vi "Inverter Command Write.vi"(0 "GEA2 Reference In":refnum<k24>, 5 "Command Requested":T5, 7 "Command Inputs":T3={"Stop"={"Command Requested"=enum."2 - Stop", "Command Sequence #"=0}, "Closed Loop Spin"={"Command Requested"=enum."4 - Closed Loop", "Command Sequence #"=0, "Closed Loop Ramp Rate"=0, "Closed Loop Target Speed"=0}, "Dry Load Sense"={"Command Requested"=enum."4 - Closed Loop", "Command Sequence #"=0, "Dry Load Ramp Rate 1"=0, "Dry Load Target Speed 1"=0, "Dry Load Dwell Time"=0, "Dry Load Dwell Sample #"=0, "Dry Load Ramp Rate 2"=0, "Dry Load Target Speed 2"=0, "DryLoad Dwell Period(Msec)"=0, "DryLoad Ramp Sample(Msec)"=0}, "Agitate"={"Command Sequence #"=0, "Agitate # of Entries"=0, "Agitate Repeat Count"=0, "Agitate Ramp Rate 1"=0, "Agitate Target Speed 1"=0, "Agitate On Time(Msec) 1"=0, "Agitate Off Time(Msec) 1"=0, "Agitate Ramp Rate 2"=0, "Agitate Target Speed 2"=0, "Agitate On Time(Msec) 2"=0, "Agitate Off Time(Msec) 2"=0, "Agitate Ramp Rate 3"=0, "Agitate Target Speed 3"=0, "Agitate On Time(Msec) 3"=0, "Agitate Off Time(Msec) 3"=0, "Agitate Ramp Rate 4"=0, "Agitate Target Speed 4"=0, "Agitate On Time(Msec) 4"=0, "Agitate Off Time(Msec) 4"=0, "Agitate Ramp Rate 5"=0, "Agitate Target Speed 5"=0, "Agitate On Time(Msec) 5"=0, "Agitate Off Time(Msec) 5"=0, "Agitate Ramp Rate 6"=0, "Agitate Target Speed 6"=0, "Agitate On Time(Msec) 6"=0, "Agitate Off Time(Msec) 6"=0, "Agitate Ramp Rate 7"=0, "Agitate Target Speed 7"=0, "Agitate On Time(Msec) 7"=0, "Agitate Off Time(Msec) 7"=0, "Agitate Ramp Rate 8"=0, "Agitate Target Speed 8"=0, "Agitate On Time(Msec) 8"=0, "Agitate Off Time(Msec) 8"=0, "Agitate Ramp Rate 9"=0, "Agitate Target Speed 9"=0, "Agitate On Time(Msec) 9"=0, "Agitate Off Time(Msec) 9"=0, "Agitate Ramp Rate 10"=0, "Agitate Target Speed 10"=0, "Agitate On Time(Msec) 10"=0, "Agitate Off Time(Msec) 10"=0, "Entry 1"=FALSE, "Entry 2"=FALSE, "Entry 3"=FALSE, "Entry 4"=FALSE, "Entry 5"=FALSE, "Entry 6"=FALSE, "Entry 7"=FALSE, "Entry 8"=FALSE, "Entry 9"=FALSE, "Entry 10"=FALSE, "Command Requested"=enum."3 - Agitate"}, "Open Loop"={"Command Sequence #"=0, "Open Loop # of Entries "=0, "Open Loop Repeat Count"=0, "Open Loop Amplitude % 1"=0, "Open Loop Target Speed 1"=0, "Open Loop On time(Msec) 1"=0, "Open Loop Off Time(Msec) 1"=0, "Open Loop Amplitude % 2"=0, "Open Loop Target Speed 2"=0, "Open Loop On time(Msec) 2"=0, "Open Loop Off Time(Msec) 2"=0, "Open Loop Amplitude % 3"=0, "Open Loop Target Speed 3"=0, "Open Loop On time(Msec) 3"=0, "Open Loop Off Time(Msec) 3"=0, "Open Loop Amplitude % 4"=0, "Open Loop Target Speed 4"=0, "Open Loop On time(Msec) 4"=0, "Open Loop Off Time(Msec) 4"=0, "Open Loop Amplitude % 5"=0, "Open Loop Target Speed 5"=0, "Open Loop On time(Msec) 5"=0, "Open Loop Off Time(Msec) 5"=0, "Open Loop Amplitude % 6"=0, "Open Loop Target Speed 6"=0, "Open Loop On time(Msec) 6"=0, "Open Loop Off Time(Msec) 6"=0, "Open Loop Amplitude % 7"=0, "Open Loop Target Speed 7"=0, "Open Loop On time(Msec) 7"=0, "Open Loop Off Time(Msec) 7"=0, "Open Loop Amplitude % 8"=0, "Open Loop Target Speed 8"=0, "Open Loop On time(Msec) 8"=0, "Open Loop Off Time(Msec) 8"=0, "Open Loop Amplitude % 9"=0, "Open Loop Target Speed 9"=0, "Open Loop On time(Msec) 9"=0, "Open Loop Off Time(Msec) 9"=0, "Open Loop Amplitude % 10"=0, "Open Loop Target Speed 10"=0, "Open Loop On time(Msec) 10"=0, "Open Loop Off Time(Msec) 10"=0, "Entry 1"=FALSE, "Entry 2"=FALSE, "Entry 3"=FALSE, "Entry 4"=FALSE, "Entry 5"=FALSE, "Entry 6"=FALSE, "Entry 7"=FALSE, "Entry 8"=FALSE, "Entry 9"=FALSE, "Entry 10"=FALSE, "Command Requested"=enum."5 - Open Loop"}, "Do Nothing"={"Command Requested"=enum."1 - Do Nothing", "Command Sequence #"=255}, "Invalid Command"={"Command Requested"=enum."0 - Invalid Command", "Command Sequence #"=255}} {"Open Loop"."Open Loop # of Entries" max=10; "Agitate"."Agitate # of Entries" max=10}, 11 "Error In":errorcluster) -> (4 "GEA2 Reference Out":refnum<k24>, 6 "appended array":T1[](array[typedef]) {"ERD Number" format="%.0x"}, 15 "Error Out":errorcluster)   [LabVIEW 2021]
uses:
  D:/Common/LabVIEW GEA2 Toolkit/source/GEA3 DLL Source/GeaCommunication.dll
  Common/LabVIEW GEA2 Toolkit/source/GEA3 DLL Source/GeaCommunication.dll
  Type Defs/Command Requested.ctl
  Type Defs/Command Inputs.ctl
  Laundry Tool (TLMB)/Laundry Tool (TLMB)/Laundry Tool Support/type defs/Inverter_Stop.ctl
  Laundry Tool (TLMB)/Laundry Tool (TLMB)/Laundry Tool Support/type defs/Inverter_Closed_Loop_Spin.ctl
  Laundry Tool (TLMB)/Laundry Tool (TLMB)/Laundry Tool Support/type defs/Inverter_Dry_Load_Sense.ctl
  Laundry Tool (TLMB)/Laundry Tool (TLMB)/Laundry Tool Support/type defs/Inverter_Agitate.ctl
  Laundry Tool (TLMB)/Laundry Tool (TLMB)/Laundry Tool Support/type defs/Inverter_Open_Loop.ctl
  Laundry Tool (TLMB)/Laundry Tool (TLMB)/Laundry Tool Support/type defs/Inverter_Do_Nothing.ctl
  Laundry Tool (TLMB)/Laundry Tool (TLMB)/Laundry Tool Support/type defs/Inverter_Invalid_command.ctl
  Common/LabVIEW GEA2 Toolkit/GEA3/type defs/ERD Write Data In.ctl
  Common/LabVIEW GEA2 Toolkit/GEA3/type defs/Data Type.ctl
  Common/LabVIEW GEA2 Toolkit/GEA3/type defs/Source_Destination.ctl
  Common/LabVIEW GEA2 Toolkit/GEA3/library/GEA2_Toolkit.lvlib
panel:
  in  "Standalone?":bool
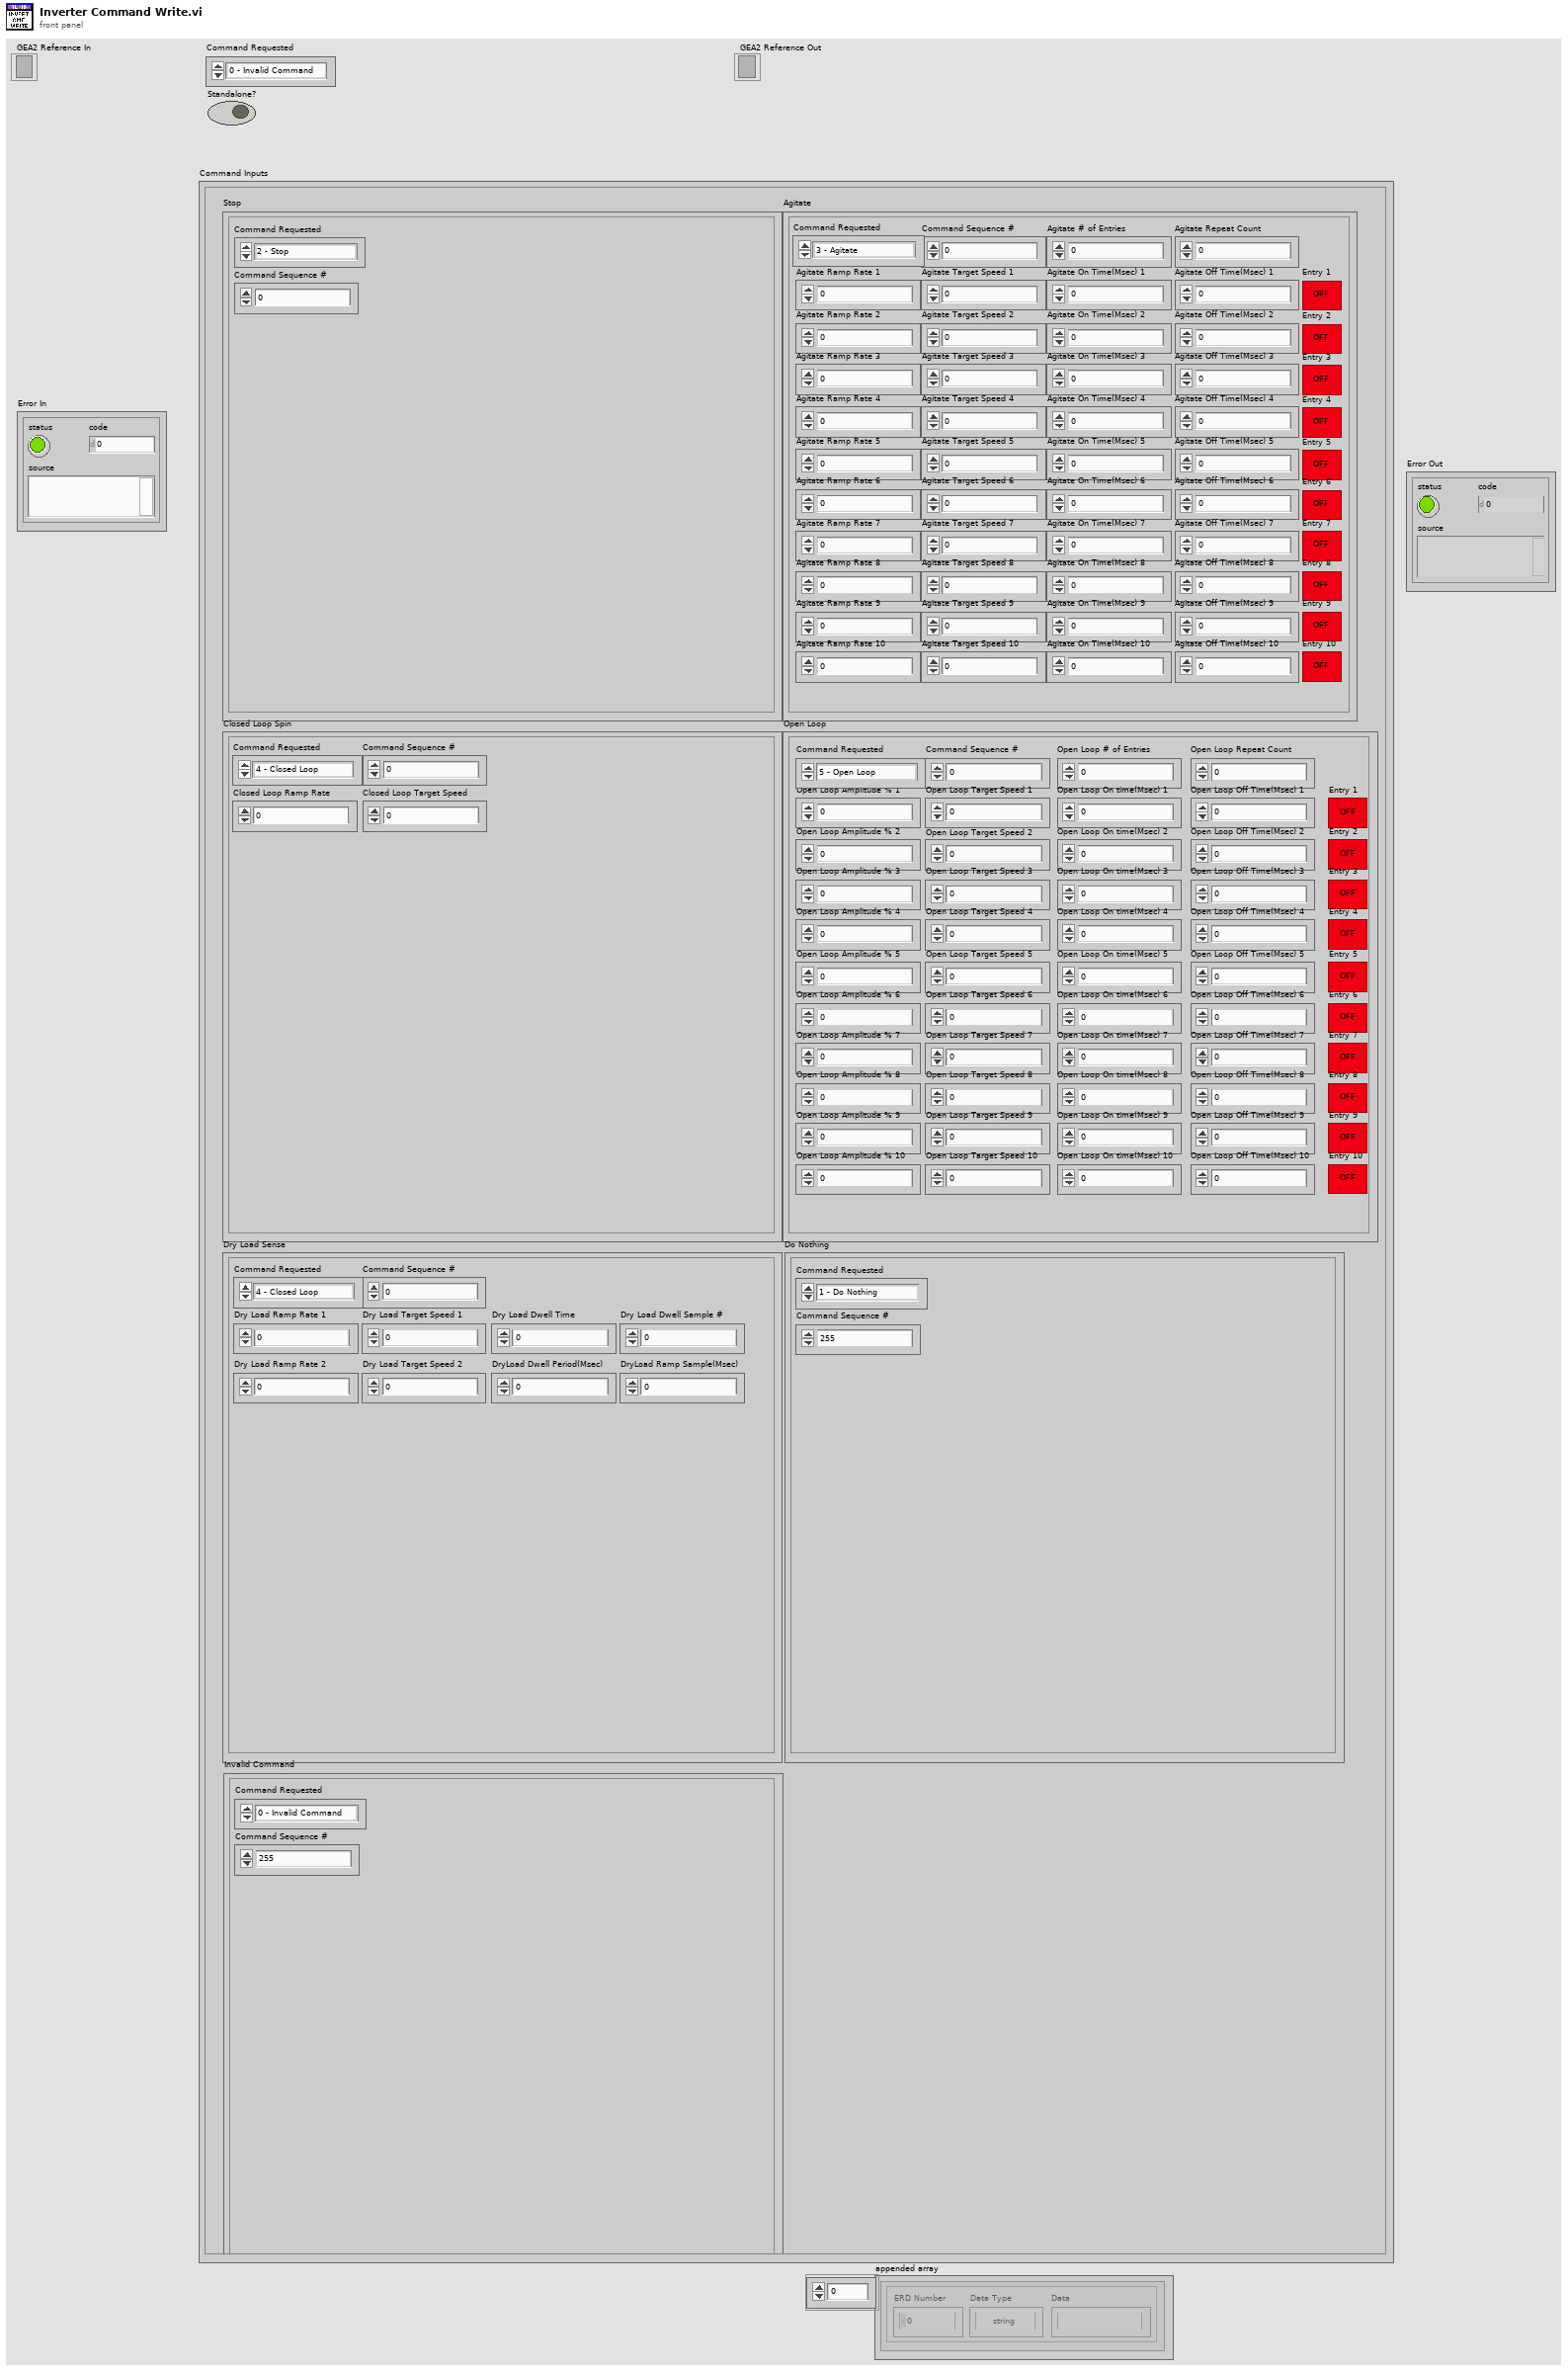
[diagram p1: front panel]
types:
  T1 = typedef "ERD Write Data In.ctl" = cluster{"ERD Number":u16, "Data Type":T2, "Data":string}
  T2 = typedef "Data Type.ctl" = enum16{"string", "boolean", "uint8_t", "uint16_t", "uint32_t", "uint64_t", "int8_t", "int16_t", "int32_t", "int64_t"}
  T3 = typedef "Command Inputs.ctl" = cluster{"Stop":T4, "Closed Loop Spin":T6, "Dry Load Sense":T7, "Agitate":T8, "Open Loop":T9, "Do Nothing":T10, "Invalid Command":T11}
  T4 = typedef "Inverter_Stop.ctl" = cluster{"Command Requested":T5, "Command Sequence #":u8}
  T5 = typedef "Command Requested.ctl" = enum16{"0 - Invalid Command", "1 - Do Nothing", "2 - Stop", "3 - Agitate", "4 - Closed Loop", "5 - Open Loop", "6 - Dry Load Sense"}
  T6 = typedef "Inverter_Closed_Loop_Spin.ctl" = cluster{"Command Requested":T5, "Command Sequence #":u8, "Closed Loop Ramp Rate":u16, "Closed Loop Target Speed":i16}
  T7 = typedef "Inverter_Dry_Load_Sense.ctl" = cluster{"Command Requested":T5, "Command Sequence #":u8, "Dry Load Ramp Rate 1":u16, "Dry Load Target Speed 1":i16, "Dry Load Dwell Time":u16, "Dry Load Dwell Sample #":u16, "Dry Load Ramp Rate 2":u16, "Dry Load Target Speed 2":i16, "DryLoad Dwell Period(Msec)":u16, "DryLoad Ramp Sample(Msec)":u16}
  T8 = typedef "Inverter_Agitate.ctl" = cluster{"Command Sequence #":u8, "Agitate # of Entries":u8, "Agitate Repeat Count":u8, "Agitate Ramp Rate 1":u16, "Agitate Target Speed 1":i16, "Agitate On Time(Msec) 1":u16, "Agitate Off Time(Msec) 1":u16, "Agitate Ramp Rate 2":u16, "Agitate Target Speed 2":i16, "Agitate On Time(Msec) 2":u16, "Agitate Off Time(Msec) 2":u16, "Agitate Ramp Rate 3":u16, "Agitate Target Speed 3":i16, "Agitate On Time(Msec) 3":u16, "Agitate Off Time(Msec) 3":u16, "Agitate Ramp Rate 4":u16, "Agitate Target Speed 4":i16, "Agitate On Time(Msec) 4":u16, "Agitate Off Time(Msec) 4":u16, "Agitate Ramp Rate 5":u16, "Agitate Target Speed 5":i16, "Agitate On Time(Msec) 5":u16, "Agitate Off Time(Msec) 5":u16, "Agitate Ramp Rate 6":u16, "Agitate Target Speed 6":i16, "Agitate On Time(Msec) 6":u16, "Agitate Off Time(Msec) 6":u16, "Agitate Ramp Rate 7":u16, "Agitate Target Speed 7":i16, "Agitate On Time(Msec) 7":u16, "Agitate Off Time(Msec) 7":u16, "Agitate Ramp Rate 8":u16, "Agitate Target Speed 8":i16, "Agitate On Time(Msec) 8":u16, "Agitate Off Time(Msec) 8":u16, "Agitate Ramp Rate 9":u16, "Agitate Target Speed 9":i16, "Agitate On Time(Msec) 9":u16, "Agitate Off Time(Msec) 9":u16, "Agitate Ramp Rate 10":u16, "Agitate Target Speed 10":i16, "Agitate On Time(Msec) 10":u16, "Agitate Off Time(Msec) 10":u16, "Entry 1":bool, "Entry 2":bool, "Entry 3":bool, "Entry 4":bool, "Entry 5":bool, "Entry 6":bool, "Entry 7":bool, "Entry 8":bool, "Entry 9":bool, "Entry 10":bool, "Command Requested":T5}
  T9 = typedef "Inverter_Open_Loop.ctl" = cluster{"Command Sequence #":u8, "Open Loop # of Entries ":u8, "Open Loop Repeat Count":u8, "Open Loop Amplitude % 1":i16, "Open Loop Target Speed 1":i16, "Open Loop On time(Msec) 1":u16, "Open Loop Off Time(Msec) 1":u16, "Open Loop Amplitude % 2":i16, "Open Loop Target Speed 2":i16, "Open Loop On time(Msec) 2":u16, "Open Loop Off Time(Msec) 2":u16, "Open Loop Amplitude % 3":i16, "Open Loop Target Speed 3":i16, "Open Loop On time(Msec) 3":u16, "Open Loop Off Time(Msec) 3":u16, "Open Loop Amplitude % 4":i16, "Open Loop Target Speed 4":i16, "Open Loop On time(Msec) 4":u16, "Open Loop Off Time(Msec) 4":u16, "Open Loop Amplitude % 5":i16, "Open Loop Target Speed 5":i16, "Open Loop On time(Msec) 5":u16, "Open Loop Off Time(Msec) 5":u16, "Open Loop Amplitude % 6":i16, "Open Loop Target Speed 6":i16, "Open Loop On time(Msec) 6":u16, "Open Loop Off Time(Msec) 6":u16, "Open Loop Amplitude % 7":i16, "Open Loop Target Speed 7":i16, "Open Loop On time(Msec) 7":u16, "Open Loop Off Time(Msec) 7":u16, "Open Loop Amplitude % 8":i16, "Open Loop Target Speed 8":i16, "Open Loop On time(Msec) 8":u16, "Open Loop Off Time(Msec) 8":u16, "Open Loop Amplitude % 9":i16, "Open Loop Target Speed 9":i16, "Open Loop On time(Msec) 9":u16, "Open Loop Off Time(Msec) 9":u16, "Open Loop Amplitude % 10":i16, "Open Loop Target Speed 10":i16, "Open Loop On time(Msec) 10":u16, "Open Loop Off Time(Msec) 10":u16, "Entry 1":bool, "Entry 2":bool, "Entry 3":bool, "Entry 4":bool, "Entry 5":bool, "Entry 6":bool, "Entry 7":bool, "Entry 8":bool, "Entry 9":bool, "Entry 10":bool, "Command Requested":T5}
  T10 = typedef "Inverter_Do_Nothing.ctl" = cluster{"Command Requested":T5, "Command Sequence #":u8}
  T11 = typedef "Inverter_Invalid_command.ctl" = cluster{"Command Requested":T5, "Command Sequence #":u8}
  T12 = typedef "Source_Destination.ctl" = cluster{"Source":u8, "Destination":u8}
  T13 = typedef "Data In.ctl" = cluster{"Source":u8, "Destination":u8, "Command":u8, "Message":string}
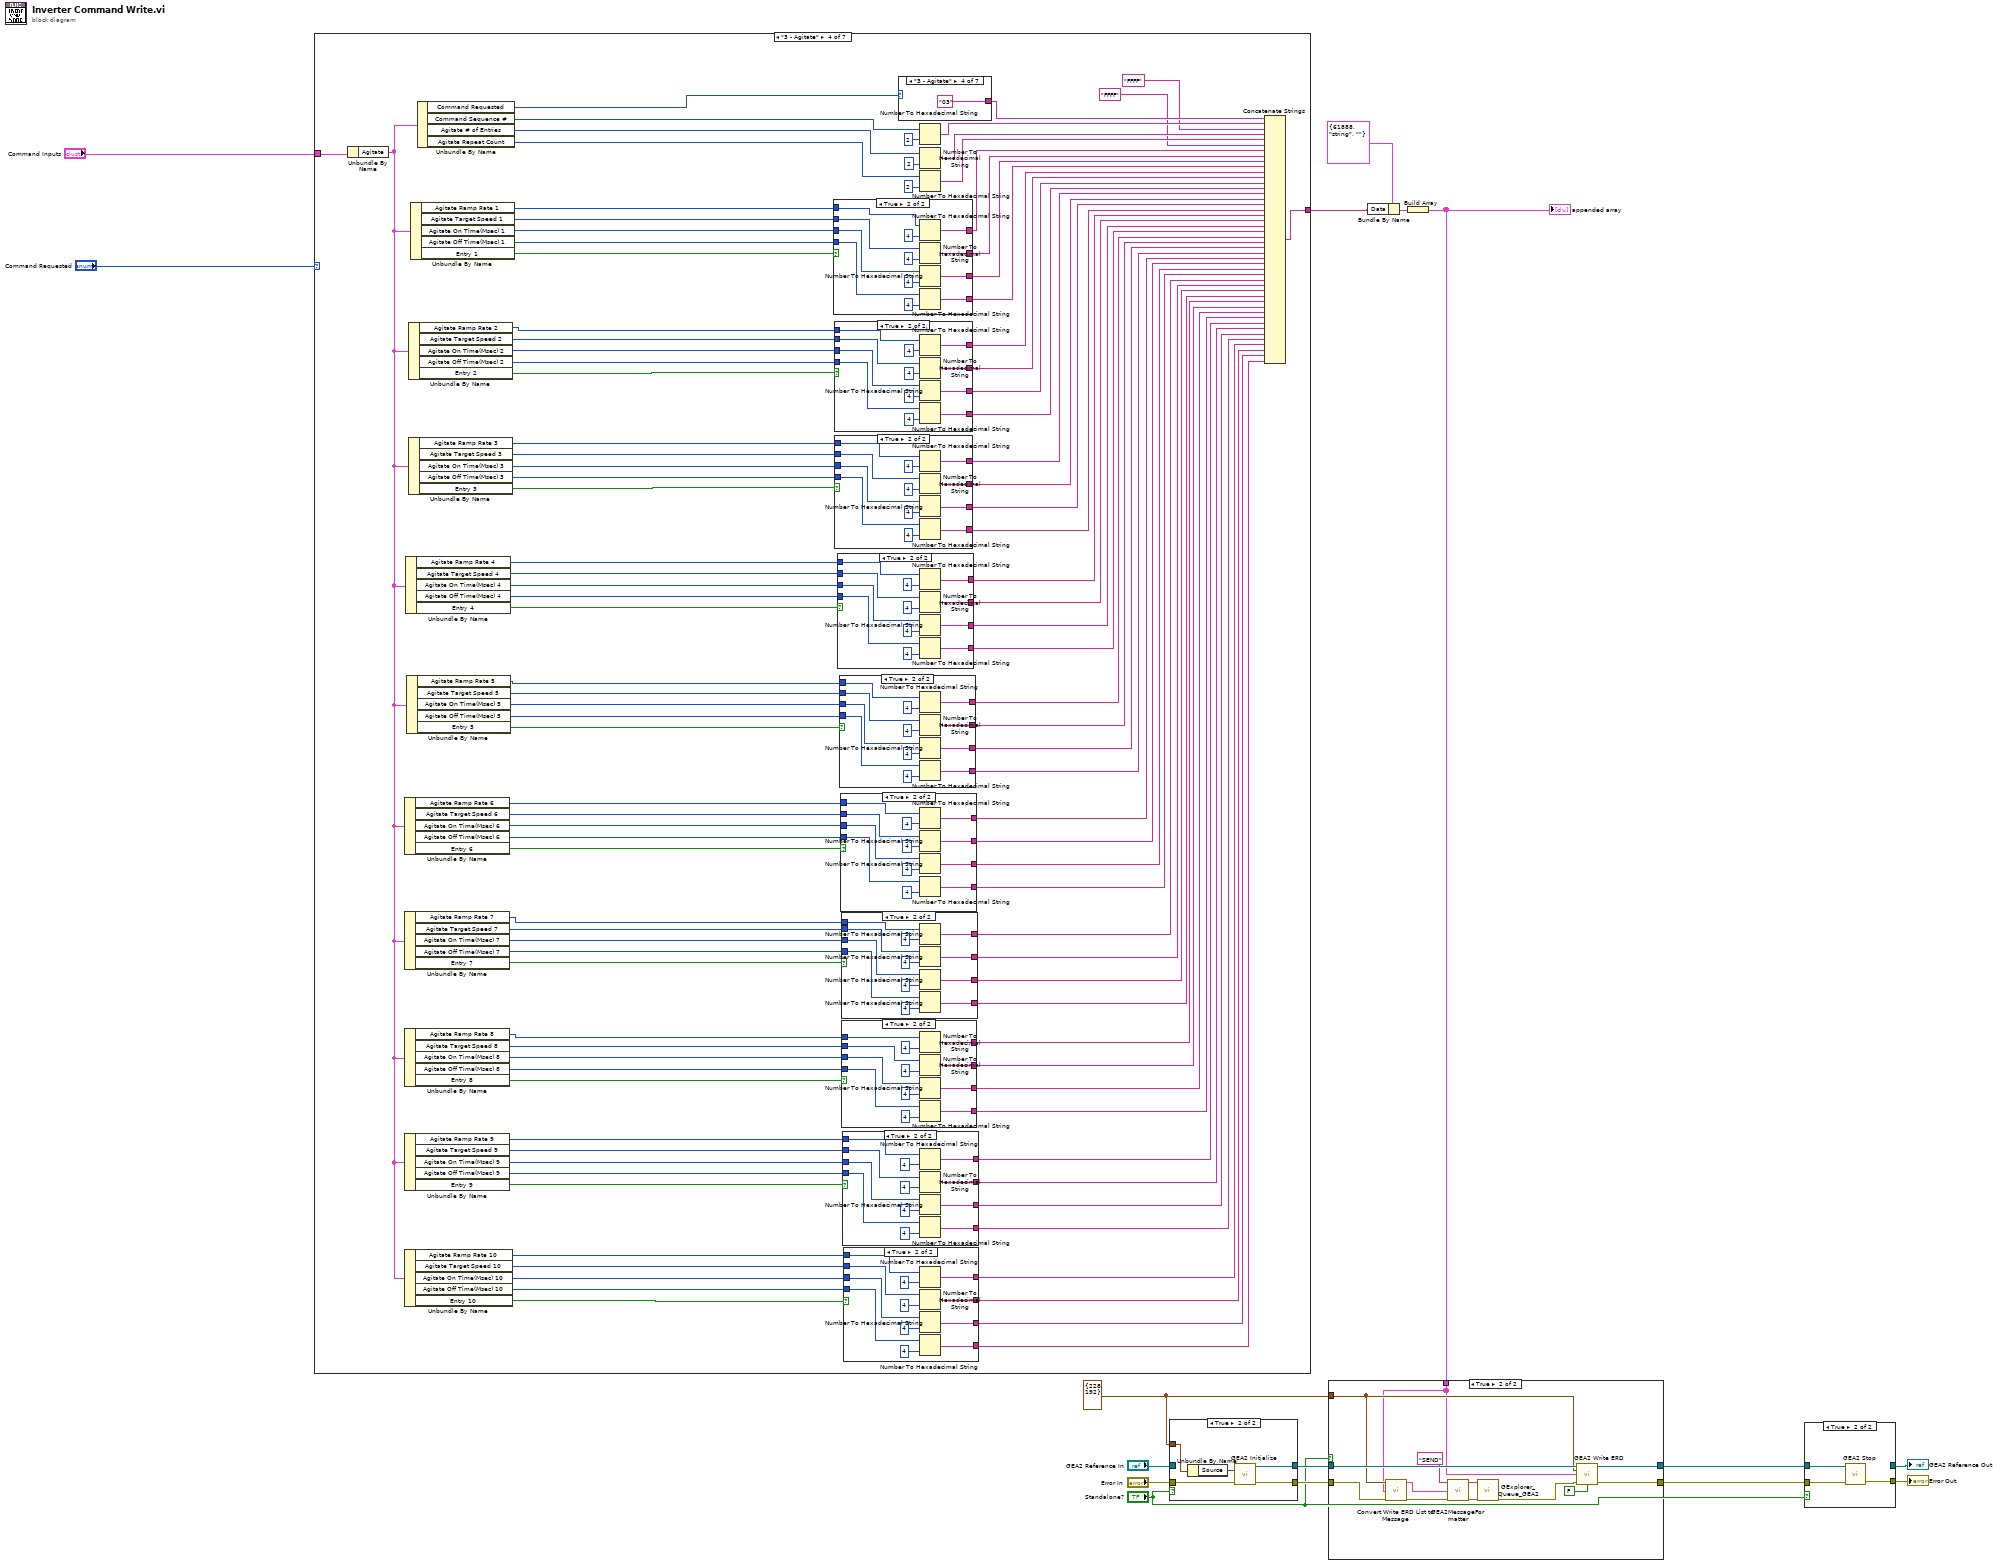
[diagram p0: block diagram]
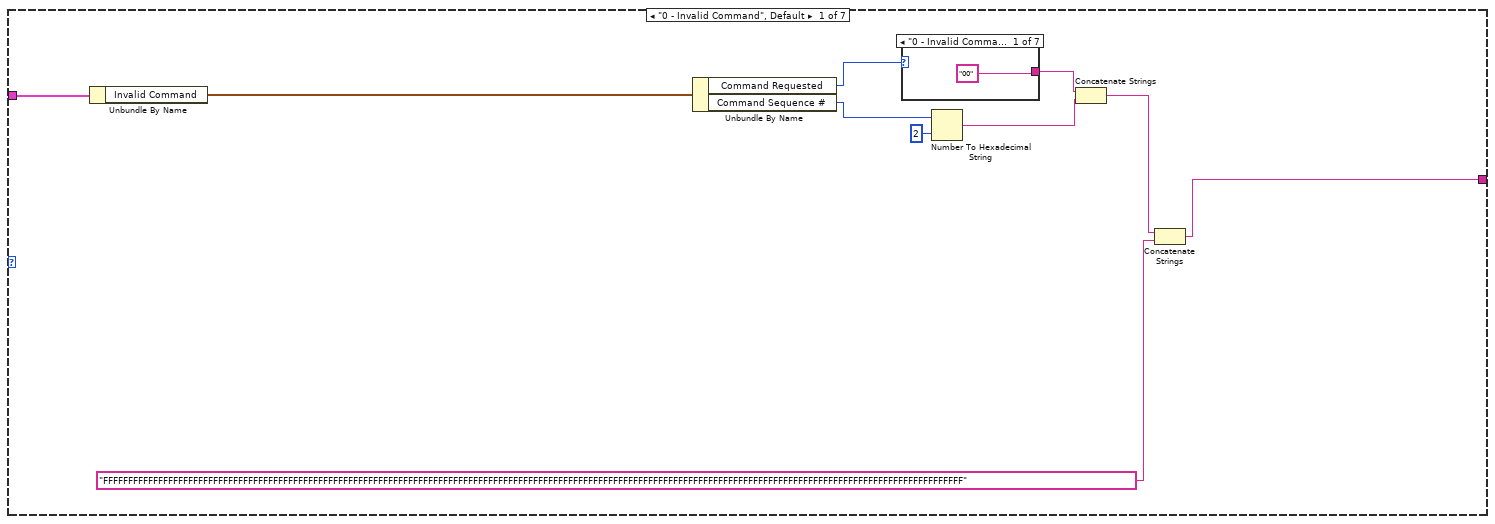
[diagram p5: hidden frame]
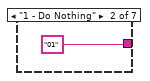
[diagram p6: hidden frame]
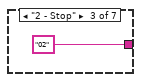
[diagram p7: hidden frame]
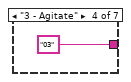
[diagram p8: hidden frame]
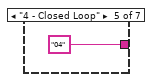
[diagram p9: hidden frame]
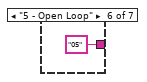
[diagram p10: hidden frame]
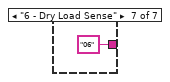
[diagram p11: hidden frame]
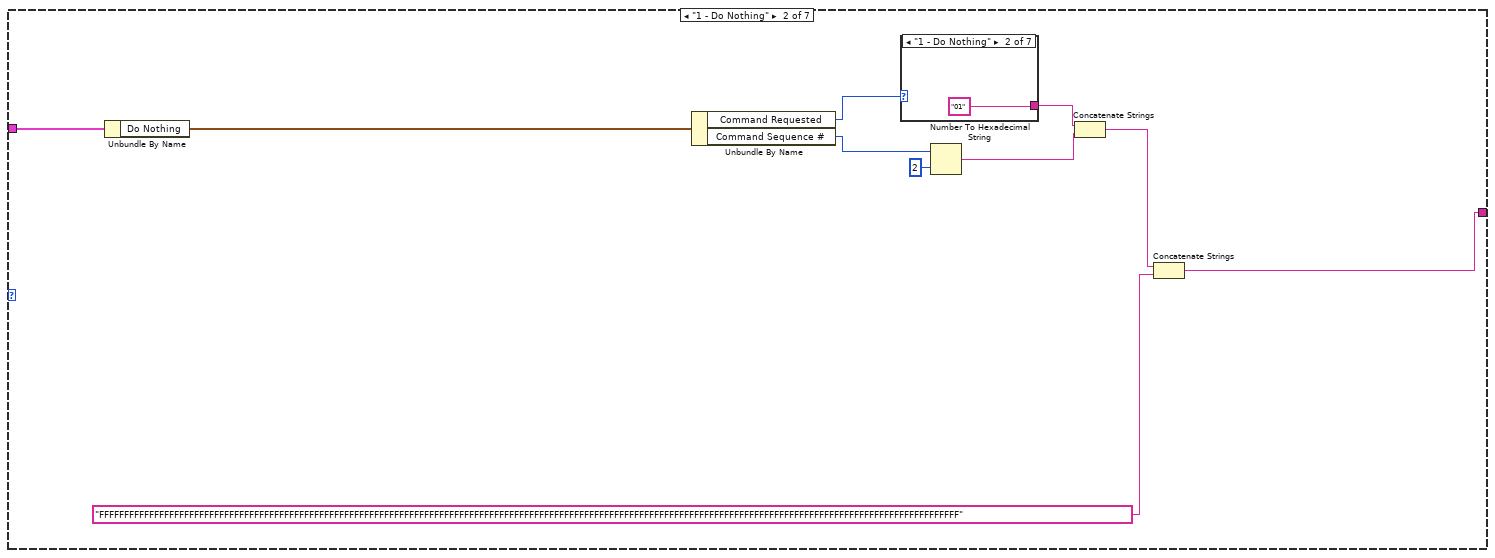
[diagram p12: hidden frame]
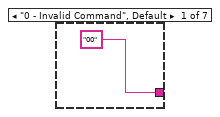
[diagram p13: hidden frame]
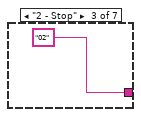
[diagram p14: hidden frame]
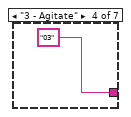
[diagram p15: hidden frame]
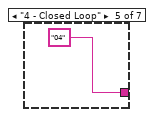
[diagram p16: hidden frame]
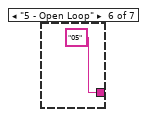
[diagram p17: hidden frame]
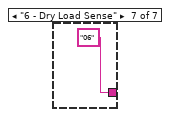
[diagram p18: hidden frame]
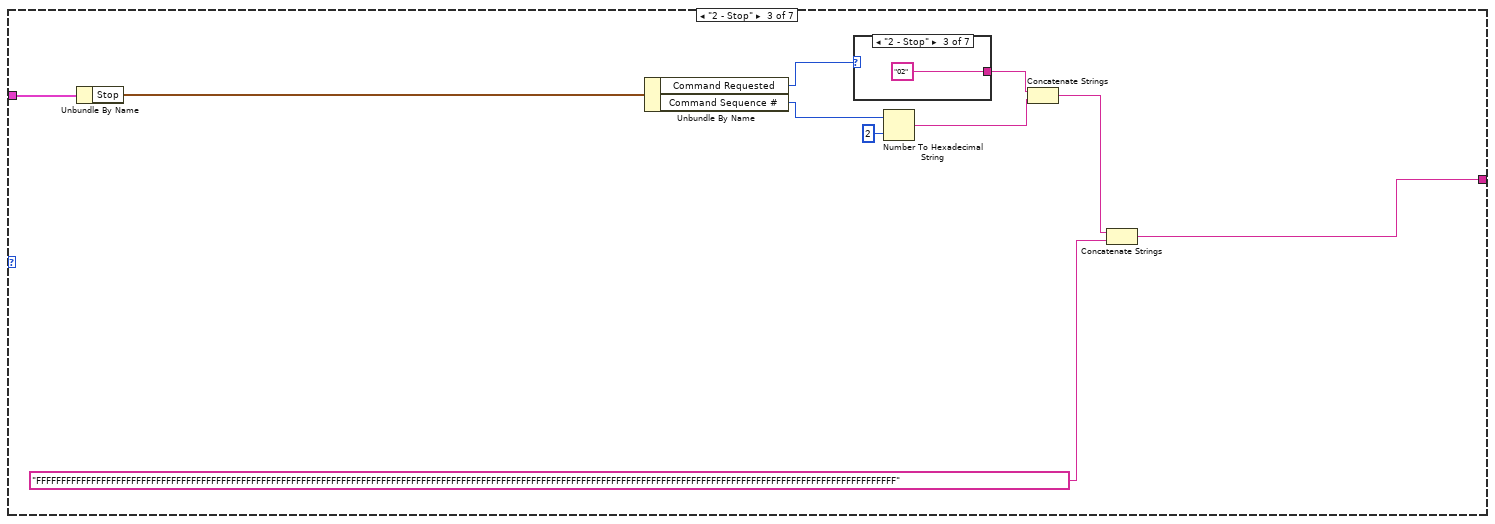
[diagram p19: hidden frame]
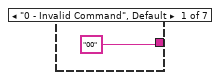
[diagram p20: hidden frame]
diagram:
  w6 = T12 {"Source"=228, "Destination"=192} ("GEA Inputs")
  n1 = case shown="\"3 - Agitate\"" "Command Requested" {
    tunnel: [w17 w34 w51 w121 w341 w415 w637] -> w2
    tunnel: "Command Inputs" -> [w18 w35 w52 w120 w342 w416 w638]
    frame "0 - Invalid Command", Default {
      n2 = Unbundle By Name(w18) -> ("Invalid Command"=w19:T11)
      n3 = Unbundle By Name(w19) -> ("Command Requested"=w26:T5, "Command Sequence #"=w25:u8)
      n4 = case shown="\"0 - Invalid Command\", Default" w26 {
        tunnel: ["00" "01" "02" "03" "04" "05" "06"] -> w23
        frame "0 - Invalid Command", Default {
        }
        frame "1 - Do Nothing" {
        }
        frame "2 - Stop" {
        }
        frame "3 - Agitate" {
        }
        frame "4 - Closed Loop" {
        }
        frame "5 - Open Loop" {
        }
        frame "6 - Dry Load Sense" {
        }
      }
      n5 = Number To Hexadecimal String(1:i16 2 ("width (-)"), 2:w25) -> (0:w22:string)
      n6 = Concatenate Strings(w23, w22) -> (w21:string)
      n7 = Concatenate Strings(w21, "FFFFFFFFFFFFFFFFFFFFFFFFFFFFFFFFFFFFFFFFFFFFFFFFFFFFFFFFFFFFFFFFFFFFFFFFFFFFFFFFFFFFFFFFFFFFFFFFFFFFFFFFFFFFFFFFFFFFFFFFFFFFFFFFFFFFFFFFFFFFFFFFFFFFFFFFFFFFFFFFFFFFFFFFFFFF" ("string")) -> (w17:string)
    }
    frame "1 - Do Nothing" {
      n8 = Unbundle By Name(w35) -> ("Do Nothing"=w36:T10)
      n9 = Unbundle By Name(w36) -> ("Command Requested"=w43:T5, "Command Sequence #"=w42:u8)
      n10 = case shown="\"1 - Do Nothing\"" w43 {
        tunnel: ["00" "01" "02" "03" "04" "05" "06"] -> w40
        frame "0 - Invalid Command", Default {
        }
        frame "1 - Do Nothing" {
        }
        frame "2 - Stop" {
        }
        frame "3 - Agitate" {
        }
        frame "4 - Closed Loop" {
        }
        frame "5 - Open Loop" {
        }
        frame "6 - Dry Load Sense" {
        }
      }
      n11 = Number To Hexadecimal String(1:i16 2 ("width (-)"), 2:w42) -> (0:w39:string)
      n12 = Concatenate Strings(w40, w39) -> (w38:string)
      n13 = Concatenate Strings(w38, "FFFFFFFFFFFFFFFFFFFFFFFFFFFFFFFFFFFFFFFFFFFFFFFFFFFFFFFFFFFFFFFFFFFFFFFFFFFFFFFFFFFFFFFFFFFFFFFFFFFFFFFFFFFFFFFFFFFFFFFFFFFFFFFFFFFFFFFFFFFFFFFFFFFFFFFFFFFFFFFFFFFFFFFFFFFF" ("string")) -> (w34:string)
    }
    frame "2 - Stop" {
      n14 = Unbundle By Name(w52) -> ("Stop"=w53:T4)
      n15 = Unbundle By Name(w53) -> ("Command Requested"=w60:T5, "Command Sequence #"=w59:u8)
      n16 = case shown="\"2 - Stop\"" w60 {
        tunnel: ["00" "01" "02" "03" "04" "05" "06"] -> w57
        frame "0 - Invalid Command", Default {
        }
        frame "1 - Do Nothing" {
        }
        frame "2 - Stop" {
        }
        frame "3 - Agitate" {
        }
        frame "4 - Closed Loop" {
        }
        frame "5 - Open Loop" {
        }
        frame "6 - Dry Load Sense" {
        }
      }
      n17 = Number To Hexadecimal String(1:i16 2 ("width (-)"), 2:w59) -> (0:w56:string)
      n18 = Concatenate Strings(w57, w56) -> (w55:string)
      n19 = Concatenate Strings(w55, "FFFFFFFFFFFFFFFFFFFFFFFFFFFFFFFFFFFFFFFFFFFFFFFFFFFFFFFFFFFFFFFFFFFFFFFFFFFFFFFFFFFFFFFFFFFFFFFFFFFFFFFFFFFFFFFFFFFFFFFFFFFFFFFFFFFFFFFFFFFFFFFFFFFFFFFFFFFFFFFFFFFFFFFFFFFF" ("string")) -> (w51:string)
    }
    frame "3 - Agitate" {
      n20 = Unbundle By Name(w120) -> ("Agitate"=w68:T8)
      n21 = Unbundle By Name(w68) -> ("Agitate Ramp Rate 10"=w72:u16, "Agitate Target Speed 10"=w71:i16, "Agitate On Time(Msec) 10"=w70:u16, "Agitate Off Time(Msec) 10"=w69:u16, "Entry 10"=w105:bool)
      n22 = Unbundle By Name(w68) -> ("Agitate Ramp Rate 6"=w88:u16, "Agitate Target Speed 6"=w87:i16, "Agitate On Time(Msec) 6"=w86:u16, "Agitate Off Time(Msec) 6"=w85:u16, "Entry 6"=w109:bool)
      n23 = Unbundle By Name(w68) -> ("Agitate Ramp Rate 7"=w84:u16, "Agitate Target Speed 7"=w83:i16, "Agitate On Time(Msec) 7"=w82:u16, "Agitate Off Time(Msec) 7"=w81:u16, "Entry 7"=w108:bool)
      n24 = Unbundle By Name(w68) -> ("Agitate Ramp Rate 8"=w80:u16, "Agitate Target Speed 8"=w79:i16, "Agitate On Time(Msec) 8"=w78:u16, "Agitate Off Time(Msec) 8"=w77:u16, "Entry 8"=w107:bool)
      n25 = Unbundle By Name(w68) -> ("Agitate Ramp Rate 9"=w76:u16, "Agitate Target Speed 9"=w75:i16, "Agitate On Time(Msec) 9"=w74:u16, "Agitate Off Time(Msec) 9"=w73:u16, "Entry 9"=w106:bool)
      n26 = Unbundle By Name(w68) -> ("Agitate Ramp Rate 4"=w96:u16, "Agitate Target Speed 4"=w95:i16, "Agitate On Time(Msec) 4"=w94:u16, "Agitate Off Time(Msec) 4"=w93:u16, "Entry 4"=w111:bool)
      n27 = Unbundle By Name(w68) -> ("Agitate Ramp Rate 5"=w92:u16, "Agitate Target Speed 5"=w91:i16, "Agitate On Time(Msec) 5"=w90:u16, "Agitate Off Time(Msec) 5"=w89:u16, "Entry 5"=w110:bool)
      n28 = Unbundle By Name(w68) -> ("Agitate Ramp Rate 2"=w104:u16, "Agitate Target Speed 2"=w103:i16, "Agitate On Time(Msec) 2"=w102:u16, "Agitate Off Time(Msec) 2"=w101:u16, "Entry 2"=w113:bool)
      n29 = Unbundle By Name(w68) -> ("Agitate Ramp Rate 3"=w100:u16, "Agitate Target Speed 3"=w99:i16, "Agitate On Time(Msec) 3"=w98:u16, "Agitate Off Time(Msec) 3"=w97:u16, "Entry 3"=w112:bool)
      n30 = Unbundle By Name(w68) -> ("Agitate Ramp Rate 1"=w117:u16, "Agitate Target Speed 1"=w116:i16, "Agitate On Time(Msec) 1"=w115:u16, "Agitate Off Time(Msec) 1"=w114:u16, "Entry 1"=w118:bool)
      n31 = Unbundle By Name(w68) -> ("Command Requested"=w172:T5, "Command Sequence #"=w171:u8, "Agitate # of Entries"=w167:u8, "Agitate Repeat Count"=w119:u8)
      n32 = case shown="True" w118 {
        tunnel: ["FFFF" w329] -> w161
        tunnel: ["FFFF" w328] -> w160
        tunnel: ["FFFF" w327] -> w159
        tunnel: ["FFFF" w326] -> w158
        tunnel: w117 -> [_ w325]
        tunnel: w116 -> [_ w324]
        tunnel: w115 -> [_ w323]
        tunnel: w114 -> [_ w322]
        frame False {
        }
        frame True {
          n33 = Number To Hexadecimal String(1:i16 4 ("width (-)"), 2:w325) -> (0:w329:string)
          n34 = Number To Hexadecimal String(1:i16 4 ("width (-)"), 2:w324) -> (0:w328:string)
          n35 = Number To Hexadecimal String(1:i16 4 ("width (-)"), 2:w323) -> (0:w327:string)
          n36 = Number To Hexadecimal String(1:i16 4 ("width (-)"), 2:w322) -> (0:w326:string)
        }
      }
      n37 = case shown="True" w113 {
        tunnel: ["FFFF" w313] -> w157
        tunnel: ["FFFF" w312] -> w156
        tunnel: ["FFFF" w311] -> w155
        tunnel: ["FFFF" w310] -> w154
        tunnel: w104 -> [_ w309]
        tunnel: w103 -> [_ w308]
        tunnel: w102 -> [_ w307]
        tunnel: w101 -> [_ w306]
        frame False {
        }
        frame True {
          n38 = Number To Hexadecimal String(1:i16 4 ("width (-)"), 2:w309) -> (0:w313:string)
          n39 = Number To Hexadecimal String(1:i16 4 ("width (-)"), 2:w308) -> (0:w312:string)
          n40 = Number To Hexadecimal String(1:i16 4 ("width (-)"), 2:w307) -> (0:w311:string)
          n41 = Number To Hexadecimal String(1:i16 4 ("width (-)"), 2:w306) -> (0:w310:string)
        }
      }
      n42 = case shown="True" w112 {
        tunnel: ["FFFF" w297] -> w153
        tunnel: ["FFFF" w296] -> w152
        tunnel: ["FFFF" w295] -> w151
        tunnel: ["FFFF" w294] -> w150
        tunnel: w100 -> [_ w293]
        tunnel: w99 -> [_ w292]
        tunnel: w98 -> [_ w291]
        tunnel: w97 -> [_ w290]
        frame False {
        }
        frame True {
          n43 = Number To Hexadecimal String(1:i16 4 ("width (-)"), 2:w293) -> (0:w297:string)
          n44 = Number To Hexadecimal String(1:i16 4 ("width (-)"), 2:w292) -> (0:w296:string)
          n45 = Number To Hexadecimal String(1:i16 4 ("width (-)"), 2:w291) -> (0:w295:string)
          n46 = Number To Hexadecimal String(1:i16 4 ("width (-)"), 2:w290) -> (0:w294:string)
        }
      }
      n47 = case shown="True" w111 {
        tunnel: ["FFFF" w281] -> w149
        tunnel: ["FFFF" w280] -> w148
        tunnel: ["FFFF" w279] -> w147
        tunnel: ["FFFF" w278] -> w146
        tunnel: w96 -> [_ w277]
        tunnel: w95 -> [_ w276]
        tunnel: w94 -> [_ w275]
        tunnel: w93 -> [_ w274]
        frame False {
        }
        frame True {
          n48 = Number To Hexadecimal String(1:i16 4 ("width (-)"), 2:w277) -> (0:w281:string)
          n49 = Number To Hexadecimal String(1:i16 4 ("width (-)"), 2:w276) -> (0:w280:string)
          n50 = Number To Hexadecimal String(1:i16 4 ("width (-)"), 2:w275) -> (0:w279:string)
          n51 = Number To Hexadecimal String(1:i16 4 ("width (-)"), 2:w274) -> (0:w278:string)
        }
      }
      n52 = case shown="True" w110 {
        tunnel: ["FFFF" w265] -> w145
        tunnel: ["FFFF" w264] -> w144
        tunnel: ["FFFF" w263] -> w143
        tunnel: ["FFFF" w262] -> w142
        tunnel: w92 -> [_ w261]
        tunnel: w91 -> [_ w260]
        tunnel: w90 -> [_ w259]
        tunnel: w89 -> [_ w258]
        frame False {
        }
        frame True {
          n53 = Number To Hexadecimal String(1:i16 4 ("width (-)"), 2:w261) -> (0:w265:string)
          n54 = Number To Hexadecimal String(1:i16 4 ("width (-)"), 2:w260) -> (0:w264:string)
          n55 = Number To Hexadecimal String(1:i16 4 ("width (-)"), 2:w259) -> (0:w263:string)
          n56 = Number To Hexadecimal String(1:i16 4 ("width (-)"), 2:w258) -> (0:w262:string)
        }
      }
      n57 = case shown="True" w109 {
        tunnel: ["FFFF" w249] -> w141
        tunnel: ["FFFF" w248] -> w140
        tunnel: ["FFFF" w247] -> w139
        tunnel: ["FFFF" w246] -> w138
        tunnel: w88 -> [_ w245]
        tunnel: w87 -> [_ w244]
        tunnel: w86 -> [_ w243]
        tunnel: w85 -> [_ w242]
        frame False {
        }
        frame True {
          n58 = Number To Hexadecimal String(1:i16 4 ("width (-)"), 2:w245) -> (0:w249:string)
          n59 = Number To Hexadecimal String(1:i16 4 ("width (-)"), 2:w244) -> (0:w248:string)
          n60 = Number To Hexadecimal String(1:i16 4 ("width (-)"), 2:w243) -> (0:w247:string)
          n61 = Number To Hexadecimal String(1:i16 4 ("width (-)"), 2:w242) -> (0:w246:string)
        }
      }
      n62 = case shown="True" w108 {
        tunnel: ["FFFF" w233] -> w137
        tunnel: ["FFFF" w232] -> w136
        tunnel: ["FFFF" w231] -> w135
        tunnel: ["FFFF" w230] -> w134
        tunnel: w84 -> [_ w229]
        tunnel: w83 -> [_ w228]
        tunnel: w82 -> [_ w227]
        tunnel: w81 -> [_ w226]
        frame False {
        }
        frame True {
          n63 = Number To Hexadecimal String(1:i16 4 ("width (-)"), 2:w229) -> (0:w233:string)
          n64 = Number To Hexadecimal String(1:i16 4 ("width (-)"), 2:w228) -> (0:w232:string)
          n65 = Number To Hexadecimal String(1:i16 4 ("width (-)"), 2:w227) -> (0:w231:string)
          n66 = Number To Hexadecimal String(1:i16 4 ("width (-)"), 2:w226) -> (0:w230:string)
        }
      }
      n67 = case shown="True" w107 {
        tunnel: ["FFFF" w217] -> w133
        tunnel: ["FFFF" w216] -> w132
        tunnel: ["FFFF" w215] -> w131
        tunnel: ["FFFF" w214] -> w130
        tunnel: w80 -> [_ w213]
        tunnel: w79 -> [_ w212]
        tunnel: w78 -> [_ w211]
        tunnel: w77 -> [_ w210]
        frame False {
        }
        frame True {
          n68 = Number To Hexadecimal String(1:i16 4 ("width (-)"), 2:w213) -> (0:w217:string)
          n69 = Number To Hexadecimal String(1:i16 4 ("width (-)"), 2:w212) -> (0:w216:string)
          n70 = Number To Hexadecimal String(1:i16 4 ("width (-)"), 2:w211) -> (0:w215:string)
          n71 = Number To Hexadecimal String(1:i16 4 ("width (-)"), 2:w210) -> (0:w214:string)
        }
      }
      n72 = case shown="True" w106 {
        tunnel: ["FFFF" w201] -> w129
        tunnel: ["FFFF" w200] -> w128
        tunnel: ["FFFF" w199] -> w127
        tunnel: ["FFFF" w198] -> w126
        tunnel: w76 -> [_ w197]
        tunnel: w75 -> [_ w196]
        tunnel: w74 -> [_ w195]
        tunnel: w73 -> [_ w194]
        frame False {
        }
        frame True {
          n73 = Number To Hexadecimal String(1:i16 4 ("width (-)"), 2:w197) -> (0:w201:string)
          n74 = Number To Hexadecimal String(1:i16 4 ("width (-)"), 2:w196) -> (0:w200:string)
          n75 = Number To Hexadecimal String(1:i16 4 ("width (-)"), 2:w195) -> (0:w199:string)
          n76 = Number To Hexadecimal String(1:i16 4 ("width (-)"), 2:w194) -> (0:w198:string)
        }
      }
      n77 = case shown="True" w105 {
        tunnel: ["FFFF" w185] -> w125
        tunnel: ["FFFF" w184] -> w124
        tunnel: ["FFFF" w183] -> w123
        tunnel: ["FFFF" w182] -> w122
        tunnel: w72 -> [_ w181]
        tunnel: w71 -> [_ w180]
        tunnel: w70 -> [_ w179]
        tunnel: w69 -> [_ w178]
        frame False {
        }
        frame True {
          n78 = Number To Hexadecimal String(1:i16 4 ("width (-)"), 2:w181) -> (0:w185:string)
          n79 = Number To Hexadecimal String(1:i16 4 ("width (-)"), 2:w180) -> (0:w184:string)
          n80 = Number To Hexadecimal String(1:i16 4 ("width (-)"), 2:w179) -> (0:w183:string)
          n81 = Number To Hexadecimal String(1:i16 4 ("width (-)"), 2:w178) -> (0:w182:string)
        }
      }
      n82 = case shown="\"3 - Agitate\"" w172 {
        tunnel: ["00" "01" "02" "03" "04" "05" "06"] -> w170
        frame "0 - Invalid Command", Default {
        }
        frame "1 - Do Nothing" {
        }
        frame "2 - Stop" {
        }
        frame "3 - Agitate" {
        }
        frame "4 - Closed Loop" {
        }
        frame "5 - Open Loop" {
        }
        frame "6 - Dry Load Sense" {
        }
      }
      n83 = Number To Hexadecimal String(1:i16 2 ("width (-)"), 2:w171) -> (0:w169:string)
      n84 = Number To Hexadecimal String(1:i16 2 ("width (-)"), 2:w167) -> (0:w165:string)
      n85 = Number To Hexadecimal String(1:i16 2 ("width (-)"), 2:w119) -> (0:w163:string)
      n86 = Concatenate Strings(w170, w169, "FFFF" ("string"), w165, w163, "FFFF" ("string"), w161, w160, w159, w158, w157, w156, w155, w154, w153, w152, w151, w150, w149, w148, w147, w146, w145, w144, w143, w142, w141, w140, w139, w138, w137, w136, w135, w134, w133, w132, w131, w130, w129, w128, w127, w126, w125, w124, w123, w122) -> (w121:string)
    }
    frame "4 - Closed Loop" {
      n87 = Unbundle By Name(w342) -> ("Closed Loop Spin"=w346:T6)
      n88 = Unbundle By Name(w346) -> ("Command Requested"=w356:T5, "Command Sequence #"=w354:u8, "Closed Loop Ramp Rate"=w344:u16, "Closed Loop Target Speed"=w349:i16)
      n89 = case shown="\"4 - Closed Loop\"" w356 {
        tunnel: ["00" "01" "02" "03" "04" "05" "06"] -> w355
        frame "0 - Invalid Command", Default {
        }
        frame "1 - Do Nothing" {
        }
        frame "2 - Stop" {
        }
        frame "3 - Agitate" {
        }
        frame "4 - Closed Loop" {
        }
        frame "5 - Open Loop" {
        }
        frame "6 - Dry Load Sense" {
        }
      }
      n90 = Number To Hexadecimal String(1:i16 2 ("width (-)"), 2:w354) -> (0:w352:string)
      n91 = Number To Hexadecimal String(1:i16 4 ("width (-)"), 2:w344) -> (0:w345:string)
      n92 = Number To Hexadecimal String(1:i16 4 ("width (-)"), 2:w349) -> (0:w348:string)
      n93 = Concatenate Strings(w355, w352, "FFFF" ("string"), w345, w348, "FFFFFFFFFFFFFFFFFFFFFFFFFFFFFFFFFFFFFFFFFFFFFFFFFFFFFFFFFFFFFFFFFFFFFFFFFFFFFFFFFFFFFFFFFFFFFFFFFFFFFFFFFFFFFFFFFFFFFFFFFFFFFFFFFFFFFFFFFFFFFFFFFFFFFFFFFFFFFFFF") -> (w341:string)
    }
    frame "5 - Open Loop" {
      n94 = Unbundle By Name(w416) -> ("Open Loop"=w414:T9)
      n95 = Unbundle By Name(w414) -> ("Command Requested"=w466:T5, "Command Sequence #"=w465:u8, "Open Loop # of Entries"=w461:u8, "Open Loop Repeat Count"=w460:u8)
      n96 = Unbundle By Name(w414) -> ("Open Loop Amplitude % 1"=w403:i16, "Open Loop Target Speed 1"=w402:i16, "Open Loop On time(Msec) 1"=w401:u16, "Open Loop Off Time(Msec) 1"=w400:u16, "Entry 1"=w413:bool)
      n97 = Unbundle By Name(w414) -> ("Open Loop Amplitude % 2"=w399:i16, "Open Loop Target Speed 2"=w398:i16, "Open Loop On time(Msec) 2"=w397:u16, "Open Loop Off Time(Msec) 2"=w396:u16, "Entry 2"=w412:bool)
      n98 = Unbundle By Name(w414) -> ("Open Loop Amplitude % 3"=w395:i16, "Open Loop Target Speed 3"=w394:i16, "Open Loop On time(Msec) 3"=w393:u16, "Open Loop Off Time(Msec) 3"=w392:u16, "Entry 3"=w411:bool)
      n99 = Unbundle By Name(w414) -> ("Open Loop Amplitude % 4"=w391:i16, "Open Loop Target Speed 4"=w390:i16, "Open Loop On time(Msec) 4"=w389:u16, "Open Loop Off Time(Msec) 4"=w388:u16, "Entry 4"=w410:bool)
      n100 = Unbundle By Name(w414) -> ("Open Loop Amplitude % 5"=w387:i16, "Open Loop Target Speed 5"=w386:i16, "Open Loop On time(Msec) 5"=w385:u16, "Open Loop Off Time(Msec) 5"=w384:u16, "Entry 5"=w409:bool)
      n101 = Unbundle By Name(w414) -> ("Open Loop Amplitude % 6"=w383:i16, "Open Loop Target Speed 6"=w382:i16, "Open Loop On time(Msec) 6"=w381:u16, "Open Loop Off Time(Msec) 6"=w380:u16, "Entry 6"=w408:bool)
      n102 = Unbundle By Name(w414) -> ("Open Loop Amplitude % 7"=w379:i16, "Open Loop Target Speed 7"=w378:i16, "Open Loop On time(Msec) 7"=w377:u16, "Open Loop Off Time(Msec) 7"=w376:u16, "Entry 7"=w407:bool)
      n103 = Unbundle By Name(w414) -> ("Open Loop Amplitude % 8"=w375:i16, "Open Loop Target Speed 8"=w374:i16, "Open Loop On time(Msec) 8"=w373:u16, "Open Loop Off Time(Msec) 8"=w372:u16, "Entry 8"=w406:bool)
      n104 = Unbundle By Name(w414) -> ("Open Loop Amplitude % 9"=w371:i16, "Open Loop Target Speed 9"=w370:i16, "Open Loop On time(Msec) 9"=w369:u16, "Open Loop Off Time(Msec) 9"=w368:u16, "Entry 9"=w405:bool)
      n105 = Unbundle By Name(w414) -> ("Open Loop Amplitude % 10"=w367:i16, "Open Loop Target Speed 10"=w366:i16, "Open Loop On time(Msec) 10"=w365:u16, "Open Loop Off Time(Msec) 10"=w364:u16, "Entry 10"=w404:bool)
      n106 = case shown="True" w412 {
        tunnel: ["FFFF" w609] -> w452
        tunnel: ["FFFF" w608] -> w451
        tunnel: ["FFFF" w607] -> w450
        tunnel: ["FFFF" w606] -> w449
        tunnel: w399 -> [_ w605]
        tunnel: w398 -> [_ w604]
        tunnel: w397 -> [_ w603]
        tunnel: w396 -> [_ w602]
        frame False {
        }
        frame True {
          n107 = Number To Hexadecimal String(1:i16 4 ("width (-)"), 2:w605) -> (0:w609:string)
          n108 = Number To Hexadecimal String(1:i16 4 ("width (-)"), 2:w604) -> (0:w608:string)
          n109 = Number To Hexadecimal String(1:i16 4 ("width (-)"), 2:w603) -> (0:w607:string)
          n110 = Number To Hexadecimal String(1:i16 4 ("width (-)"), 2:w602) -> (0:w606:string)
        }
      }
      n111 = case shown="True" w413 {
        tunnel: ["FFFF" w625] -> w456
        tunnel: ["FFFF" w624] -> w455
        tunnel: ["FFFF" w623] -> w454
        tunnel: ["FFFF" w622] -> w453
        tunnel: w403 -> [_ w621]
        tunnel: w402 -> [_ w620]
        tunnel: w401 -> [_ w619]
        tunnel: w400 -> [_ w618]
        frame False {
        }
        frame True {
          n112 = Number To Hexadecimal String(1:i16 4 ("width (-)"), 2:w621) -> (0:w625:string)
          n113 = Number To Hexadecimal String(1:i16 4 ("width (-)"), 2:w620) -> (0:w624:string)
          n114 = Number To Hexadecimal String(1:i16 4 ("width (-)"), 2:w619) -> (0:w623:string)
          n115 = Number To Hexadecimal String(1:i16 4 ("width (-)"), 2:w618) -> (0:w622:string)
        }
      }
      n116 = case shown="True" w411 {
        tunnel: ["FFFF" w593] -> w448
        tunnel: ["FFFF" w592] -> w447
        tunnel: ["FFFF" w591] -> w446
        tunnel: ["FFFF" w590] -> w445
        tunnel: w395 -> [_ w589]
        tunnel: w394 -> [_ w588]
        tunnel: w393 -> [_ w587]
        tunnel: w392 -> [_ w586]
        frame False {
        }
        frame True {
          n117 = Number To Hexadecimal String(1:i16 4 ("width (-)"), 2:w589) -> (0:w593:string)
          n118 = Number To Hexadecimal String(1:i16 4 ("width (-)"), 2:w588) -> (0:w592:string)
          n119 = Number To Hexadecimal String(1:i16 4 ("width (-)"), 2:w587) -> (0:w591:string)
          n120 = Number To Hexadecimal String(1:i16 4 ("width (-)"), 2:w586) -> (0:w590:string)
        }
      }
      n121 = case shown="False" w410 {
        tunnel: ["FFFF" w577] -> w444
        tunnel: ["FFFF" w576] -> w443
        tunnel: ["FFFF" w575] -> w442
        tunnel: ["FFFF" w574] -> w441
        tunnel: w391 -> [_ w573]
        tunnel: w390 -> [_ w572]
        tunnel: w389 -> [_ w571]
        tunnel: w388 -> [_ w570]
        frame False {
        }
        frame True {
          n122 = Number To Hexadecimal String(1:i16 4 ("width (-)"), 2:w573) -> (0:w577:string)
          n123 = Number To Hexadecimal String(1:i16 4 ("width (-)"), 2:w572) -> (0:w576:string)
          n124 = Number To Hexadecimal String(1:i16 4 ("width (-)"), 2:w571) -> (0:w575:string)
          n125 = Number To Hexadecimal String(1:i16 4 ("width (-)"), 2:w570) -> (0:w574:string)
        }
      }
      n126 = case shown="True" w409 {
        tunnel: ["FFFF" w561] -> w440
        tunnel: ["FFFF" w560] -> w439
        tunnel: ["FFFF" w559] -> w438
        tunnel: ["FFFF" w558] -> w437
        tunnel: w387 -> [_ w557]
        tunnel: w386 -> [_ w556]
        tunnel: w385 -> [_ w555]
        tunnel: w384 -> [_ w554]
        frame False {
        }
        frame True {
          n127 = Number To Hexadecimal String(1:i16 4 ("width (-)"), 2:w557) -> (0:w561:string)
          n128 = Number To Hexadecimal String(1:i16 4 ("width (-)"), 2:w556) -> (0:w560:string)
          n129 = Number To Hexadecimal String(1:i16 4 ("width (-)"), 2:w555) -> (0:w559:string)
          n130 = Number To Hexadecimal String(1:i16 4 ("width (-)"), 2:w554) -> (0:w558:string)
        }
      }
      n131 = case shown="True" w408 {
        tunnel: ["FFFF" w545] -> w436
        tunnel: ["FFFF" w544] -> w435
        tunnel: ["FFFF" w543] -> w434
        tunnel: ["FFFF" w542] -> w433
        tunnel: w383 -> [_ w541]
        tunnel: w382 -> [_ w540]
        tunnel: w381 -> [_ w539]
        tunnel: w380 -> [_ w538]
        frame False {
        }
        frame True {
          n132 = Number To Hexadecimal String(1:i16 4 ("width (-)"), 2:w541) -> (0:w545:string)
          n133 = Number To Hexadecimal String(1:i16 4 ("width (-)"), 2:w540) -> (0:w544:string)
          n134 = Number To Hexadecimal String(1:i16 4 ("width (-)"), 2:w539) -> (0:w543:string)
          n135 = Number To Hexadecimal String(1:i16 4 ("width (-)"), 2:w538) -> (0:w542:string)
        }
      }
      n136 = case shown="True" w407 {
        tunnel: ["FFFF" w529] -> w432
        tunnel: ["FFFF" w528] -> w431
        tunnel: ["FFFF" w527] -> w430
        tunnel: ["FFFF" w526] -> w429
        tunnel: w379 -> [_ w525]
        tunnel: w378 -> [_ w524]
        tunnel: w377 -> [_ w523]
        tunnel: w376 -> [_ w522]
        frame False {
        }
        frame True {
          n137 = Number To Hexadecimal String(1:i16 4 ("width (-)"), 2:w525) -> (0:w529:string)
          n138 = Number To Hexadecimal String(1:i16 4 ("width (-)"), 2:w524) -> (0:w528:string)
          n139 = Number To Hexadecimal String(1:i16 4 ("width (-)"), 2:w523) -> (0:w527:string)
          n140 = Number To Hexadecimal String(1:i16 4 ("width (-)"), 2:w522) -> (0:w526:string)
        }
      }
      n141 = case shown="True" w406 {
        tunnel: ["FFFF" w513] -> w428
        tunnel: ["FFFF" w512] -> w427
        tunnel: ["FFFF" w511] -> w426
        tunnel: ["FFFF" w510] -> w425
        tunnel: w375 -> [_ w509]
        tunnel: w374 -> [_ w508]
        tunnel: w373 -> [_ w507]
        tunnel: w372 -> [_ w506]
        frame False {
        }
        frame True {
          n142 = Number To Hexadecimal String(1:i16 4 ("width (-)"), 2:w509) -> (0:w513:string)
          n143 = Number To Hexadecimal String(1:i16 4 ("width (-)"), 2:w508) -> (0:w512:string)
          n144 = Number To Hexadecimal String(1:i16 4 ("width (-)"), 2:w507) -> (0:w511:string)
          n145 = Number To Hexadecimal String(1:i16 4 ("width (-)"), 2:w506) -> (0:w510:string)
        }
      }
      n146 = case shown="True" w405 {
        tunnel: ["FFFF" w497] -> w424
        tunnel: ["FFFF" w496] -> w423
        tunnel: ["FFFF" w495] -> w422
        tunnel: ["FFFF" w494] -> w421
        tunnel: w371 -> [_ w493]
        tunnel: w370 -> [_ w492]
        tunnel: w369 -> [_ w491]
        tunnel: w368 -> [_ w490]
        frame False {
        }
        frame True {
          n147 = Number To Hexadecimal String(1:i16 4 ("width (-)"), 2:w493) -> (0:w497:string)
          n148 = Number To Hexadecimal String(1:i16 4 ("width (-)"), 2:w492) -> (0:w496:string)
          n149 = Number To Hexadecimal String(1:i16 4 ("width (-)"), 2:w491) -> (0:w495:string)
          n150 = Number To Hexadecimal String(1:i16 4 ("width (-)"), 2:w490) -> (0:w494:string)
        }
      }
      n151 = case shown="True" w404 {
        tunnel: ["FFFF" w481] -> w420
        tunnel: ["FFFF" w480] -> w419
        tunnel: ["FFFF" w479] -> w418
        tunnel: ["FFFF" w478] -> w417
        tunnel: w367 -> [_ w477]
        tunnel: w366 -> [_ w476]
        tunnel: w365 -> [_ w475]
        tunnel: w364 -> [_ w474]
        frame False {
        }
        frame True {
          n152 = Number To Hexadecimal String(1:i16 4 ("width (-)"), 2:w477) -> (0:w481:string)
          n153 = Number To Hexadecimal String(1:i16 4 ("width (-)"), 2:w476) -> (0:w480:string)
          n154 = Number To Hexadecimal String(1:i16 4 ("width (-)"), 2:w475) -> (0:w479:string)
          n155 = Number To Hexadecimal String(1:i16 4 ("width (-)"), 2:w474) -> (0:w478:string)
        }
      }
      n156 = case shown="\"5 - Open Loop\"" w466 {
        tunnel: ["00" "01" "02" "03" "04" "05" "06"] -> w464
        frame "0 - Invalid Command", Default {
        }
        frame "1 - Do Nothing" {
        }
        frame "2 - Stop" {
        }
        frame "3 - Agitate" {
        }
        frame "4 - Closed Loop" {
        }
        frame "5 - Open Loop" {
        }
        frame "6 - Dry Load Sense" {
        }
      }
      n157 = Number To Hexadecimal String(1:i16 2 ("width (-)"), 2:w465) -> (0:w463:string)
      n158 = Number To Hexadecimal String(1:i16 2 ("width (-)"), 2:w461) -> (0:w459:string)
      n159 = Number To Hexadecimal String(1:i16 2 ("width (-)"), 2:w460) -> (0:w458:string)
      n160 = Concatenate Strings(w464, w463, "FFFF" ("string"), w459, w458, "FFFF" ("string"), w456, w455, w454, w453, w452, w451, w450, w449, w448, w447, w446, w445, w444, w443, w442, w441, w440, w439, w438, w437, w436, w435, w434, w433, w432, w431, w430, w429, w428, w427, w426, w425, w424, w423, w422, w421, w420, w419, w418, w417) -> (w415:string)
    }
    frame "6 - Dry Load Sense" {
      # "2"
      n161 = Unbundle By Name(w638) -> ("Dry Load Sense"=w665:T7)
      n162 = Unbundle By Name(w665) -> ("Command Requested"=w669:T5, "Command Sequence #"=w668:u8, "Dry Load Ramp Rate 1"=w662:u16, "Dry Load Target Speed 1"=w659:i16, "Dry Load Dwell Time"=w656:u16, "Dry Load Dwell Sample #"=w653:u16, "DryLoad Dwell Period(Msec)"=w650:u16, "Dry Load Ramp Rate 2"=w648:u16, "Dry Load Target Speed 2"=w646:i16, "DryLoad Ramp Sample(Msec)"=w644:u16)
      n163 = case shown="\"6 - Dry Load Sense\"" w669 {
        tunnel: ["00" "01" "02" "03" "04" "05" "06"] -> w670
        frame "0 - Invalid Command", Default {
        }
        frame "1 - Do Nothing" {
        }
        frame "2 - Stop" {
        }
        frame "3 - Agitate" {
        }
        frame "4 - Closed Loop" {
        }
        frame "5 - Open Loop" {
        }
        frame "6 - Dry Load Sense" {
        }
      }
      n164 = Number To Hexadecimal String(1:i16 2 ("width (-)"), 2:w668) -> (0:w666:string)
      n165 = Number To Hexadecimal String(1:i16 4 ("width (-)"), 2:w662) -> (0:w661:string)
      n166 = Number To Hexadecimal String(1:i16 4 ("width (-)"), 2:w659) -> (0:w658:string)
      n167 = Number To Hexadecimal String(1:i16 4 ("width (-)"), 2:w656) -> (0:w655:string)
      n168 = Number To Hexadecimal String(1:i16 4 ("width (-)"), 2:w653) -> (0:w652:string)
      n169 = Number To Hexadecimal String(1:i16 4 ("width (-)"), 2:w650) -> (0:w649:string)
      n170 = Number To Hexadecimal String(1:i16 4 ("width (-)"), 2:w648) -> (0:w642:string)
      n171 = Number To Hexadecimal String(1:i16 4 ("width (-)"), 2:w646) -> (0:w641:string)
      n172 = Number To Hexadecimal String(1:i16 4 ("width (-)"), 2:w644) -> (0:w640:string)
      n173 = Concatenate Strings(w670, w666, "FFFF" ("string"), w661, w658, w655, w652, w649, w642, w641, w640, "FFFFFFFFFFFFFFFFFFFFFFFFFFFFFFFFFFFFFFFFFFFFFFFFFFFFFFFFFFFFFFFFFFFFFFFFFFFFFFFFFFFFFFFFFFFFFFFFFFFFFFFFFFFFFFFFFFFFFFFFFFFFFFFFFFFFFFFF") -> (w637:string)
    }
  }
  n174 = case shown="True" "Standalone?" {
    tunnel: w6 -> [_ w680]
    tunnel: [w679 w683] -> w11
    tunnel: [w678 w682] -> w4
    tunnel: "Error In" -> [w678 w681]
    tunnel: "GEA2 Reference In" -> [w679 _]
    frame False {
    }
    frame True {
      n175 = Unbundle By Name(w680) -> ("Source"=w684:u8)
      n176 = call "GEA2 Initialize.vi"("Source Address"=w684, "error in"=w681) -> ("GEA2 Reference Out"=w683:refnum<k24>, "error out"=w682:errorcluster)  [unwired: 11 in, 1 out]
    }
  }
  n177 = Bundle By Name(cluster=T1 {"ERD Number"=61888, "Data Type"=enum."string", "Data"=""} ("ERD Write Data In"), "Data"=w2) -> (w15:T1)
  n178 = Build Array(w15) -> (w5:T1[])
  "appended array" <- w5
  n179 = case shown="True" "Standalone?" {
    tunnel: w11 -> [w686 w699]
    tunnel: [w686 w698] -> w10
    tunnel: [w685 w697] -> w9
    tunnel: w6 -> [_ w690]
    tunnel: w5 -> [_ w689]
    tunnel: w4 -> [w685 w688]
    frame False {
    }
    frame True {
      n180 = call "Convert Write ERD List to Message.vi"("GEA Inputs"=w690, "Write ERD List"=w689, "Error In"=w688) -> ("GEA Message"=w691:T13, "Error Out"=w693:errorcluster)  [unwired: 11 in]
      n181 = call "GEA2MessageFormatter.vi"("Prefix(Send/Recv)"="SEND", "GEA2 Data In"=w691, "Error In"=w693) -> ("Output String"=w694:string, "Error Out"=w695:errorcluster)  [unwired: 11 in]
      n182 = call "GExplorer_Queue_GEA2.vi"("Output String"=w694, "error in (no error)"=w695) -> ("error out"=w687:errorcluster)  [unwired: 13 in]
      n183 = call "GEA2 Write ERD.vi"("GEA2 Reference In"=w699, "GEA Inputs"=w690, "Write ERD List"=w689, "Error In"=w687, "Verify ERD Response?"=FALSE) -> ("GEA2 Reference Out"=w698:refnum<k24>, "Error Out"=w697:errorcluster)  [unwired: 8 in, 1 out]
    }
  }
  n184 = case shown="True" "Standalone?" {
    tunnel: w9 -> [w701 w704]
    tunnel: w10 -> [w700 w703]
    tunnel: [w701 w702] -> w7
    tunnel: [w700 _] -> w8
    frame False {
    }
    frame True {
      n185 = call "GEA2 Stop.vi"("GEA2 Reference In"=w703, "Error In"=w704) -> ("Error Out"=w702:errorcluster)  [unwired: 13 in]
    }
  }
  "GEA2 Reference Out" <- w8
  "Error Out" <- w7
